vi "DaNIDemoVI_pid.vi"() -> ()   [LabVIEW 2016]
uses:
  <vilib>/userdefined/High Color/nirio_resource_hc.ctl
panel:
  out "e(n)_R":dbl(graph)
  out "I(n)_R":dbl(graph)
  out "I(n)_L":dbl(graph)
  out "e(n)_L":dbl(graph)
  out "Omega Left":dbl(graph)
  out "Omega Right":dbl(graph)
  in  "Ti L":dbl=1.5 format="%#_13g"
  in  "Kp L":dbl=0.03 format="%#_13g"
  in  "Td L":dbl=0.0001 format="%#_13g"
  in  "Reference L":dbl=10.0 format="%#_13g"
  in  "Kp R":dbl=0.03 format="%#_13g"
  in  "Td R":dbl=0.0001 format="%#_13g"
  in  "Ti R":dbl=1.5 format="%#_13g"
  in  "Reference R":dbl=10.0 format="%#_13g"
  in  "Mode Select":T1(ring)
  in  "IP Adress":T2="rio://169.254.0.1/RIO0"
  out "Distance Measured (m)":dbl
  in  "Servomotor Angle Offset (Degrees)":dbl
  in  "Servomotor Angle (Degrees)":dbl
  out "Rad/s Right":dbl
  out "Rad/s Left":dbl
  in  "dt (ms)":u32=65
  out "Right Motor Voltage Percentage In (-1 to 1)":dbl min=-1.0 max=1.0 step=0.01
  out "Left Motor Voltage Percentage In (-1 to 1)":dbl min=-1.0 max=1.0 step=0.01
  in  "stop":bool
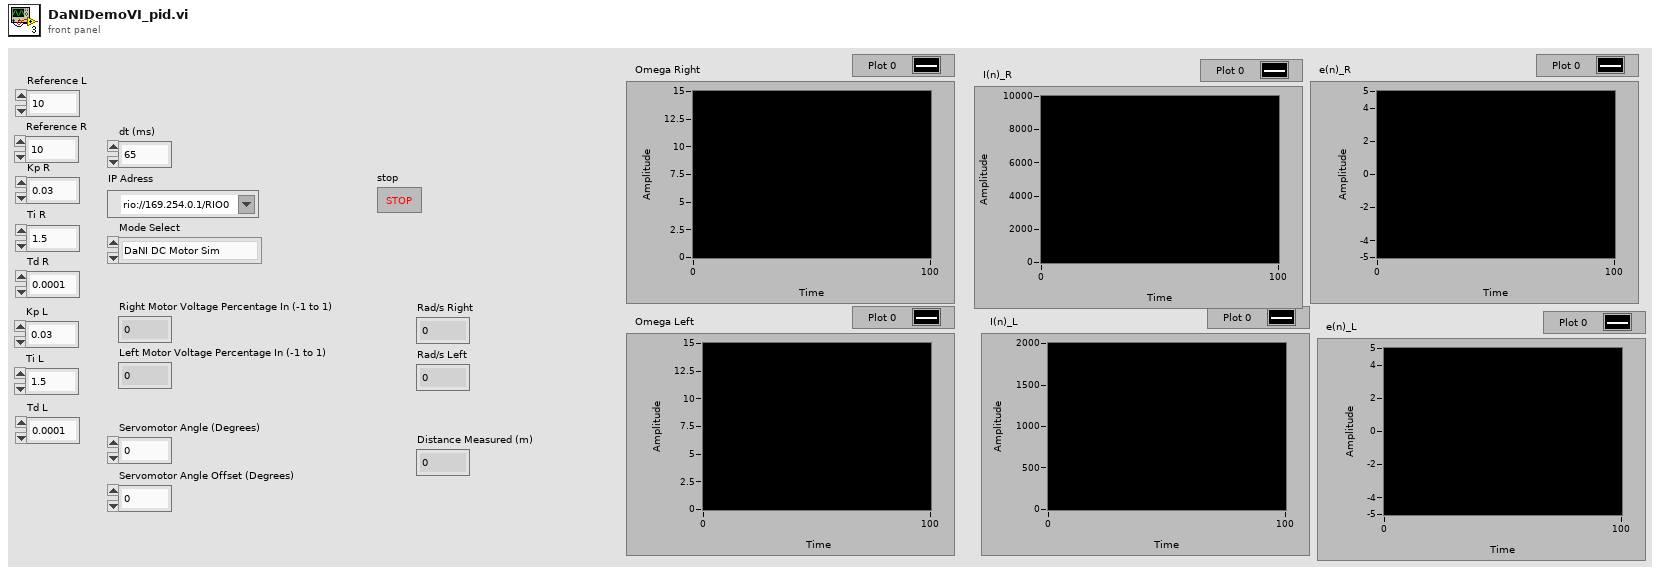
[diagram p1: front panel]
types:
  T1 = enum16{"DaNI DC Motor Sim", "DaNI Simulation", "DaNI Robot"}
  T2 = typedef "nirio_resource_hc.ctl" = tag
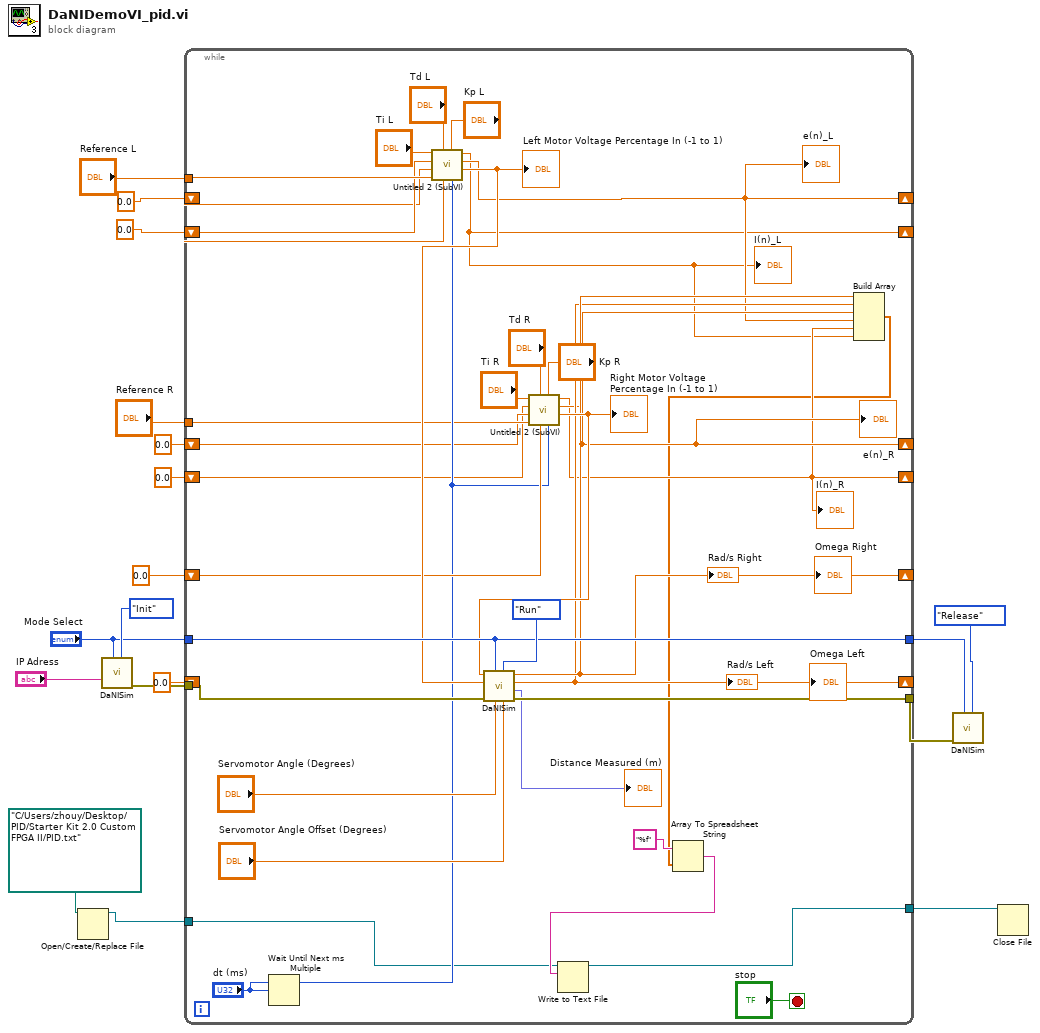
[diagram p0: block diagram]
diagram:
  n1 = Open/Create/Replace File(file path (use dialog)=path "C:/Users/zhouy/Desktop/PID/Starter Kit 2.0 Custom FPGA II/PID.txt") -> (refnum out=w2:refnum<file>)  [unwired: 5 in, 2 out]
  n2 = call "DaNISim.vi"("Action"=enum16{"Init", "Run", "Release"}."Init", "Mode Select"="Mode Select", "IP Adress"="IP Adress") -> ("error out"=w16:errorcluster)  [unwired: 5 in, 3 out]
  n3 = while {
    tunnel: w16 -> [w53]
    tunnel: "Mode Select" -> [w48]
    tunnel: [w51] -> w14
    tunnel: [w48] -> w12
    shift-right: [w25] -> _
    shift-left: 0.0 ("OmegaR") -> [w38]
    tunnel: "Reference R" -> [w32]
    shift-right: [w23] -> _
    shift-left: 0.0 ("e(n)") -> [w31]
    shift-right: [w21] -> _
    shift-left: 0.0 ("I(n)") -> [w30]
    shift-right: [w22] -> _
    shift-left: 0.0 ("e(n)") -> [w39]
    shift-right: [w24] -> _
    shift-left: 0.0 ("OmegaL") -> [w41]
    shift-right: [w20] -> _
    shift-left: 0.0 -> [w40]
    tunnel: "Reference L" -> [w42]
    tunnel: [w27] -> w3
    tunnel: w2 -> [w26]
    stop <- "stop" stop-if-true
    n4 = Wait Until Next ms Multiple(millisecond multiple="dt (ms)") -> ()  [unwired: 1 out]
    n5 = call "Untitled 2 (SubVI).vi"("dt (ms)"="dt (ms)", "Kp"="Kp L", "Omega"=w41, "Td"="Td L", "Reference"=w42, "E(n-1)"=w39, "I(n-1)"=w40, "Ti"="Ti L") -> ("u"=w43:dbl, "E(n)"=w22:dbl, "I(n)"=w20:dbl)  [unwired: 1 in]
    "Left Motor Voltage Percentage In (-1 to 1)" <- w43
    "e(n)_L" <- w22
    "I(n)_L" <- w20
    n6 = call "Untitled 2 (SubVI).vi"("dt (ms)"="dt (ms)", "Kp"="Kp R", "Omega"=w38, "Td"="Td R", "Reference"=w32, "E(n-1)"=w31, "I(n-1)"=w30, "Ti"="Ti R") -> ("u"=w37:dbl, "E(n)"=w23:dbl, "I(n)"=w21:dbl)  [unwired: 1 in]
    "Right Motor Voltage Percentage In (-1 to 1)" <- w37
    "I(n)_R" <- w21
    "e(n)_R" <- w23
    n7 = call "DaNISim.vi"("Sonar offset angle"="Servomotor Angle Offset (Degrees)", "Action"=enum16{"Init", "Run", "Release"}."Run", "Sonar angle"="Servomotor Angle (Degrees)", "Mode Select"=w48, "error in (no error)"=w53, "Ul"=w43, "Ur"=w37) -> ("error out"=w51:errorcluster, "Sonar distance"=→"Distance Measured (m)":fxp<+,32,8>, "OmegaL"=w24:dbl, "OmegaR"=w25:dbl)  [unwired: 1 in]
    "Rad/s Left" <- w24
    "Rad/s Right" <- w25
    "Omega Right" <- w25
    "Omega Left" <- w24
    n8 = Build Array(w25, w24, w23, w22, w21, w20) -> (w19:dbl[])
    n9 = Array To Spreadsheet String(array=w19, 3:"%f") -> (spreadsheet string=w28:string)  [unwired: 1 in]
    n10 = Write to Text File(file (use dialog)=w26, text=w28) -> (refnum out=w27:refnum<file>)  [unwired: 2 in, 2 out]
  }
  n11 = call "DaNISim.vi"("Action"=enum16{"Init", "Run", "Release"}."Release", "Mode Select"=w12, "error in (no error)"=w14) -> ()  [unwired: 5 in, 4 out]
  n12 = Close File(refnum=w3) -> ()  [unwired: 1 in, 2 out]
